vi "methane_reactor.vi"(3 "Dataflow In":errorcluster) -> (1 "Dataflow Out":errorcluster)   [LabVIEW 2019]
uses:
  lib/libSimulationControl/libSimulationControl.lvlib
panel:
  # "*******************************************************************\nBiogas Plant Control\n\nAuthor: Paul Zügel\nGCSC-Frankfurt am Main 2020\n\n*******************************************************************"
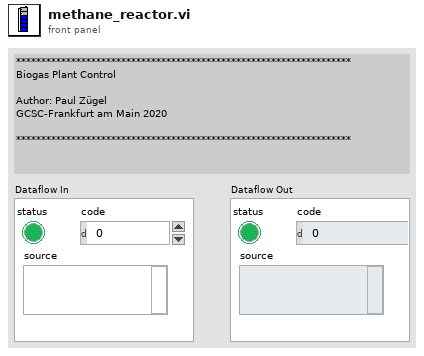
[diagram p1: front panel]
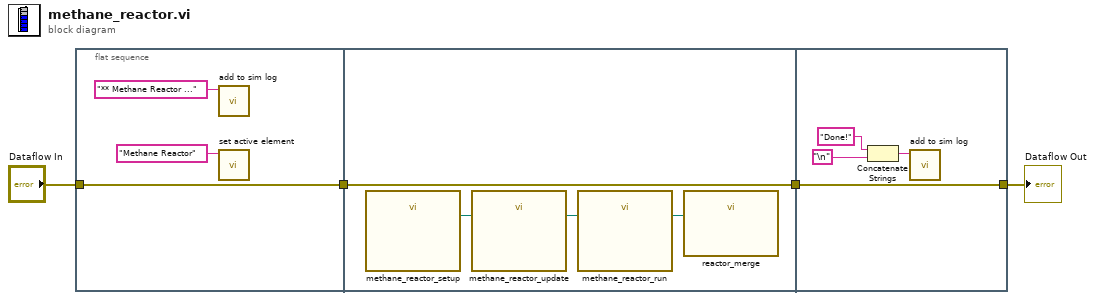
[diagram p0: block diagram]
diagram:
  n1 = flat-sequence {
    tunnel: [w7] -> w1
    tunnel: "Dataflow In" -> [w7]
    tunnel: w1 -> [w11]
    tunnel: [w11] -> w2
    tunnel: [w15] -> w3
    tunnel: w2 -> [w15]
    frame #0 {
      n2 = call "add to sim log.vi"("log"="** Methane Reactor ..." ("string")) -> ()  [unwired: 10 in, 1 out]
      n3 = call "set active element.vi"("elem"="Methane Reactor") -> ()  [unwired: 10 in, 1 out]
    }
    frame #1 {
      n4 = call "methane_reactor_setup.vi"() -> ("spec_file"=w10:path)  [unwired: 11 in]
      n5 = call "methane_reactor_update.vi"("spec_file"=w10) -> ("spec_file_dup"=w9:path)  [unwired: 10 in]
      n6 = call "methane_reactor_run.vi"("spec_file"=w9) -> ("methane_path"=w8:path)  [unwired: 10 in]
      n7 = call "reactor_merge.vi"("reactor_path"=w8) -> ()  [unwired: 11 in]
    }
    frame #2 {
      n8 = Concatenate Strings("Done!" ("string"), "\n") -> (w12:string)
      n9 = call "add to sim log.vi"("log"=w12) -> ()  [unwired: 10 in, 1 out]
    }
  }
  "Dataflow Out" <- w3
